vi "Connection Open.vi"(8 "error in (no error)":errorcluster, 11 "Connection Data In":T1) -> (0 "error out":errorcluster, 3 "Connection Data Out":T1)   [LabVIEW 2014, in "MSX-E3711_dll.lvlib"]
doc: "Abre la conexión del Web Server."
uses:
  MSX-E3711_dll.lvlib
  Typedef/Connection Data.ctl
  E:/Repositorio Magnis/INF002/v0/Modules/HAL/Drivers/Sync/ADDI-DATA MSX-E3711/API/MSXE371x.dll
  MSXE371x.dll
  E:/Repositorio Magnis/INF002/v0/Modules/HAL/Drivers/Sync/ADDI-DATA MSX-E3711/API/MXCommon.dll
  MXCommon.dll
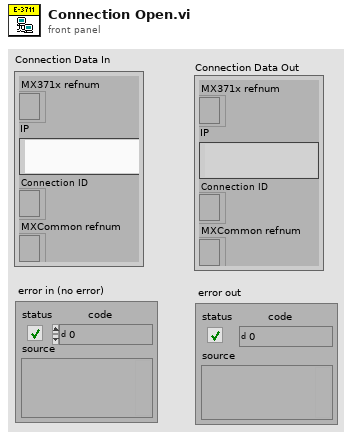
[diagram p1: front panel]
types:
  T1 = typedef "MSX-E3711_dll.lvlib/Connection Data.ctl" = cluster{"MX371x refnum":refnum<k24>, "IP":string, "Connection ID ":refnum<k5>, "MXCommon refnum":refnum<k24>}
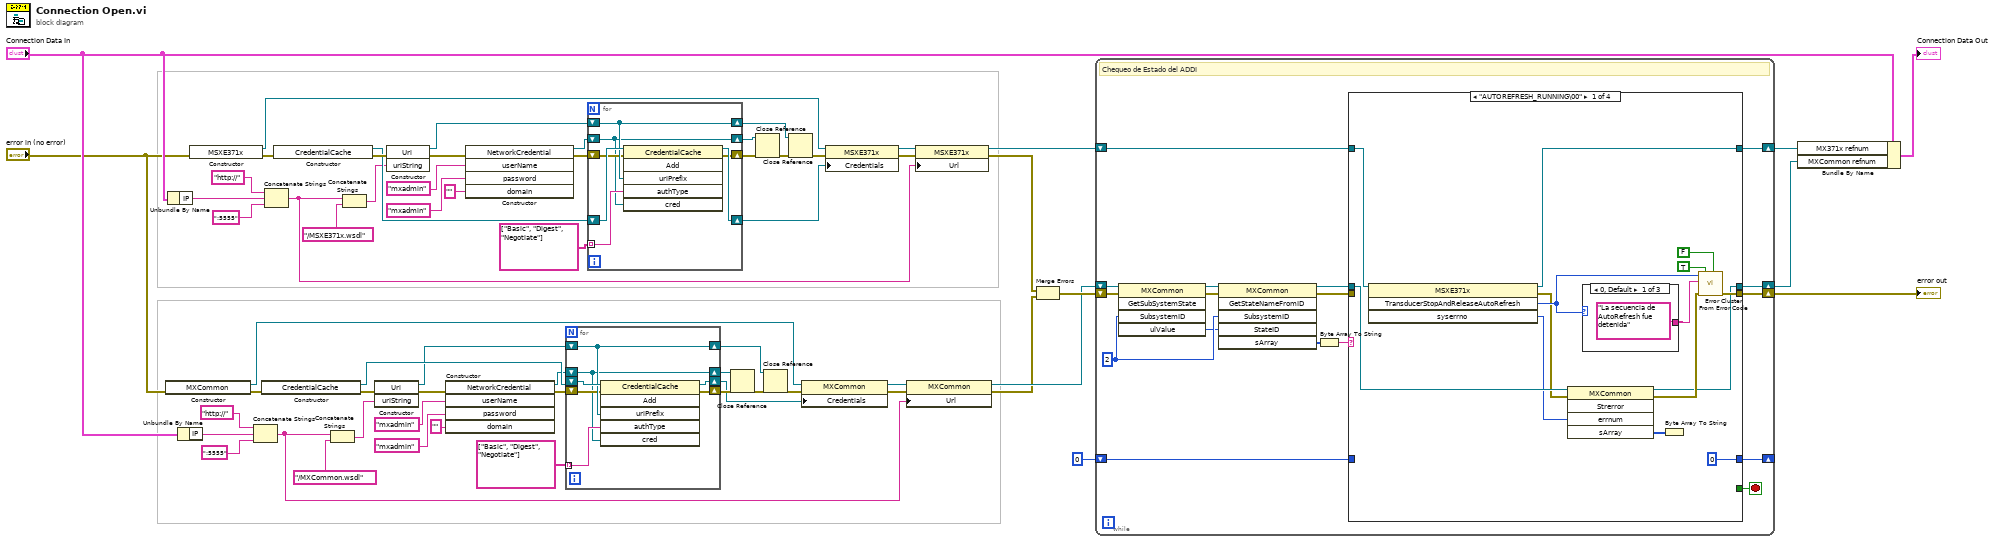
[diagram p0: block diagram]
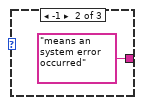
[diagram p2: hidden frame]
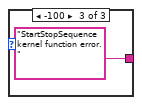
[diagram p3: hidden frame]
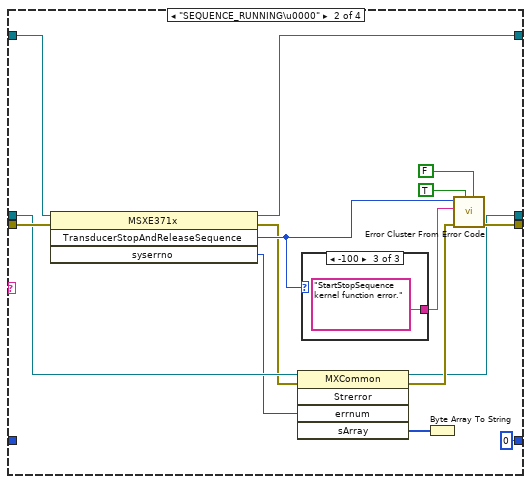
[diagram p4: hidden frame]
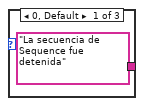
[diagram p5: hidden frame]
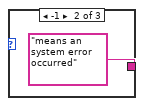
[diagram p6: hidden frame]
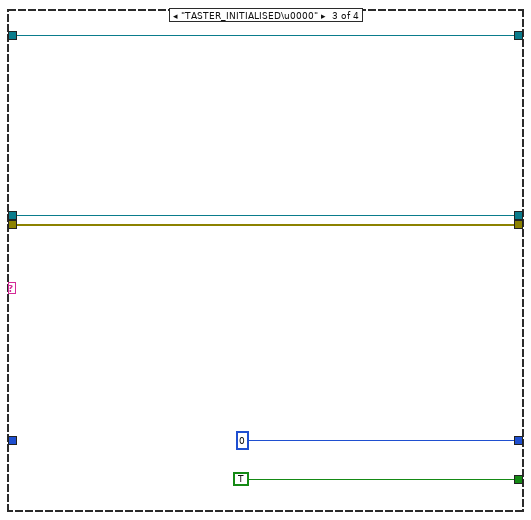
[diagram p7: hidden frame]
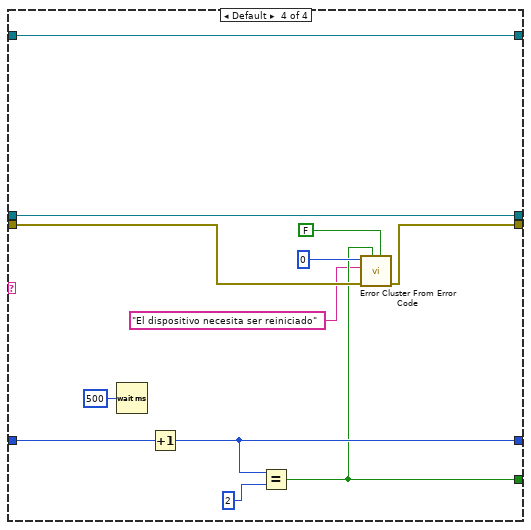
[diagram p8: hidden frame]
diagram:
  n1 = constructor class="MXCommon"(error in="error in (no error)") -> (reference out=w13:refnum<k24>, error out=w12:errorcluster)  [unwired: 2 in, 1 out]
  n2 = Unbundle By Name("Connection Data In") -> ("IP"=w45:string)
  n3 = Unbundle By Name("Connection Data In") -> ("IP"=w26:string)
  n4 = constructor class="MSXE371x"(error in="error in (no error)") -> (reference out=w5:refnum<k24>, error out=w11:errorcluster)  [unwired: 2 in, 1 out]
  n5 = Concatenate Strings("http://" ("string"), w26, ":5555" ("string")) -> (w17:string)
  n6 = constructor class="CredentialCache"(error in=w12) -> (reference out=w41:refnum<k24>, error out=w44:errorcluster)  [unwired: 2 in, 1 out]
  n7 = Concatenate Strings("http://" ("string"), w45, ":5555" ("string")) -> (w10:string)
  n8 = constructor class="CredentialCache"(error in=w11) -> (reference out=w61:refnum<k24>, error out=w64:errorcluster)  [unwired: 2 in, 1 out]
  n9 = Concatenate Strings(w17, "/MXCommon.wsdl" ("string")) -> (w28:string)
  n10 = Concatenate Strings(w10, "/MSXE371x.wsdl" ("string")) -> (w48:string)
  n11 = constructor class="Uri"(error in=w44, "uriString"=w28) -> (reference out=w40:refnum<k24>, error out=w43:errorcluster)  [unwired: 2 in, 2 out]
  n12 = constructor class="Uri"(error in=w64, "uriString"=w48) -> (reference out=w60:refnum<k24>, error out=w63:errorcluster)  [unwired: 2 in, 2 out]
  n13 = constructor class="NetworkCredential"(error in=w43, "userName"="mxadmin", "password"="mxadmin" ("userName"), "domain"="" ("userName")) -> (reference out=w39:refnum<k24>, error out=w38:errorcluster)  [unwired: 2 in, 4 out]
  n14 = constructor class="NetworkCredential"(error in=w63, "userName"="mxadmin", "password"="mxadmin" ("userName"), "domain"="" ("userName")) -> (reference out=w59:refnum<k24>, error out=w58:errorcluster)  [unwired: 2 in, 4 out]
  n15 = for {
    tunnel: string[] ["Basic", "Digest", "Negotiate"] -> [w66] mode=indexing
    shift-right: [w67] -> w34
    shift-left: w38 -> [w68]
    shift-right: [w70] -> w36
    shift-left: w40 -> [w70]
    shift-right: [w69] -> w20
    shift-left: w41 -> [w71]
    shift-right: [w65] -> w37
    shift-left: w39 -> [w65]
    n16 = invoke class="CredentialCache" method="Add"(reference=w71, error in=w68, "uriPrefix"=w70, "authType"=w66, "cred"=w65) -> (reference out=w69:refnum<k24>, error out=w67:errorcluster)  [unwired: 1 in, 4 out]
  }
  n17 = for {
    tunnel: string[] ["Basic", "Digest", "Negotiate"] -> [w73] mode=indexing
    shift-right: [w74] -> w54
    shift-left: w58 -> [w75]
    shift-right: [w77] -> w56
    shift-left: w60 -> [w77]
    shift-right: [w76] -> w3
    shift-left: w61 -> [w78]
    shift-right: [w72] -> w57
    shift-left: w59 -> [w72]
    n18 = invoke class="CredentialCache" method="Add"(reference=w78, error in=w75, "uriPrefix"=w77, "authType"=w73, "cred"=w72) -> (reference out=w76:refnum<k24>, error out=w74:errorcluster)  [unwired: 1 in, 4 out]
  }
  n19 = Close Reference(reference=w37, error in (no error)=w34) -> (error out=w35:errorcluster)
  n20 = Close Reference(reference=w57, error in (no error)=w54) -> (error out=w55:errorcluster)
  n21 = Close Reference(reference=w36, error in (no error)=w35) -> (error out=w14:errorcluster)
  n22 = Close Reference(reference=w56, error in (no error)=w55) -> (error out=w4:errorcluster)
  n23 = property class="MXCommon"(reference=w13, error in=w14, "Credentials"=w20) -> (reference out=w15:refnum<k24>, error out=w16:errorcluster)
  n24 = property class="MSXE371x"(reference=w5, error in=w4, "Credentials"=w3) -> (reference out=w7:refnum<k24>, error out=w6:errorcluster)
  n25 = property class="MXCommon"(reference=w15, error in=w16, "Url"=w17) -> (reference out=w19:refnum<k24>, error out=w18:errorcluster)
  n26 = property class="MSXE371x"(reference=w7, error in=w6, "Url"=w10) -> (reference out=w9:refnum<k24>, error out=w8:errorcluster)
  n27 = Merge Errors(w8, w18) -> (w24:errorcluster)
  n28 = while {
    shift-right: [w91] -> _
    shift-left: u32 0 ("milliseconds to wait") -> [w92]
    shift-right: [w90] -> w22
    shift-left: w19 -> [w87]
    shift-right: [w89] -> w21
    shift-left: w9 -> [w94]
    shift-right: [w88] -> w2
    shift-left: w24 -> [w86]
    stop <- w93 stop-if-true
    w85 = u64 2 ("SubsystemID 2")
    # "Chequeo de Estado del ADDI"
    n29 = invoke class="MXCommon" method="GetSubSystemState"(reference=w87, error in=w86, "SubsystemID"=w85) -> (reference out=w82:refnum<k24>, error out=w83:errorcluster, "ulValue"=w84:u64)  [unwired: 2 in, 2 out]
    n30 = invoke class="MXCommon" method="GetStateNameFromID"(reference=w82, error in=w83, "SubsystemID"=w85, "StateID"=w84) -> (reference out=w81:refnum<k24>, error out=w80:errorcluster, "sArray"=w79:u8[])  [unwired: 2 in, 3 out]
    n31 = Byte Array To String(unsigned byte array=w79) -> (string=w95:string)
    n32 = case shown="\"AUTOREFRESH_RUNNING\\00\"" w95 {
      tunnel: w94 -> [w104 w122 w131 w142]
      tunnel: w81 -> [w101 w118 w133 w143]
      tunnel: [_ _ TRUE w137] -> w93
      tunnel: w92 -> [_ _ _ w145]
      tunnel: [u32 0 u32 0 u32 0 w144] -> w91
      tunnel: [w97 w114 w133 w143] -> w90
      tunnel: [w103 w120 w131 w142] -> w89
      tunnel: w80 -> [_ w121 w132 w140]
      tunnel: [w105 w123 w132 w139] -> w88
      frame "AUTOREFRESH_RUNNING\u0000" {
        n33 = invoke class="MSXE371x" method="TransducerStopAndReleaseAutoRefresh"(reference=w104) -> (reference out=w103:refnum<k24>, error out=w100:errorcluster, "TransducerStopAndReleaseAutoRefresh"=w102:i32, "syserrno"=w99:i32)  [unwired: 3 in]
        n34 = invoke class="MXCommon" method="Strerror"(reference=w101, error in=w100, "errnum"=w99) -> (reference out=w97:refnum<k24>, error out=w98:errorcluster, "sArray"=w96:u8[])  [unwired: 2 in, 2 out]
        n35 = case shown="0, Default" w102 {
          tunnel: ["La secuencia de AutoRefresh fue detenida" "means an system error occurred" "StartStopSequence kernel function error."] -> w108
          frame 0, Default {
          }
          frame -1 {
          }
          frame -100 {
          }
        }
        n36 = Byte Array To String(unsigned byte array=w96) -> ()  [unwired: 1 out]
        n37 = call <vilib>:"Error Cluster From Error Code.vi"("is warning? (False)"=FALSE, "show call chain? (False)"=TRUE, "error in (no error)"=w98, "error message (\"\")"=w108, "error code (0)"=w102) -> ("error out"=w105:errorcluster)  [unwired: 4 in]
      }
      frame "SEQUENCE_RUNNING\u0000" {
        n38 = invoke class="MSXE371x" method="TransducerStopAndReleaseSequence"(reference=w122, error in=w121) -> (reference out=w120:refnum<k24>, error out=w117:errorcluster, "TransducerStopAndReleaseSequence"=w119:i32, "syserrno"=w116:i32)  [unwired: 2 in]
        n39 = invoke class="MXCommon" method="Strerror"(reference=w118, error in=w117, "errnum"=w116) -> (reference out=w114:refnum<k24>, error out=w115:errorcluster, "sArray"=w113:u8[])  [unwired: 2 in, 2 out]
        n40 = case shown="-100" w119 {
          tunnel: ["La secuencia de Sequence fue detenida" "means an system error occurred" "StartStopSequence kernel function error."] -> w126
          frame 0, Default {
          }
          frame -1 {
          }
          frame -100 {
          }
        }
        n41 = Byte Array To String(unsigned byte array=w113) -> ()  [unwired: 1 out]
        n42 = call <vilib>:"Error Cluster From Error Code.vi"("is warning? (False)"=FALSE, "show call chain? (False)"=TRUE, "error in (no error)"=w115, "error message (\"\")"=w126, "error code (0)"=w119) -> ("error out"=w123:errorcluster)  [unwired: 4 in]
      }
      frame "TASTER_INITIALISED\u0000" {
      }
      frame Default {
        n43 = Wait (ms)(milliseconds to wait=u32 500) -> ()  [unwired: 1 out]
        n44 = Increment(x=w145) -> (x+1=w144:u32)
        n45 = Equal?(x=w144, y=u32 2 ("milliseconds to wait")) -> (x = y?=w137:bool)
        n46 = call <vilib>:"Error Cluster From Error Code.vi"("is warning? (False)"=FALSE, "show call chain? (False)"=w137, "error in (no error)"=w140, "error message (\"\")"="El dispositivo necesita ser reiniciado", "error code (0)"=0) -> ("error out"=w139:errorcluster)  [unwired: 4 in]
      }
    }
  }
  "error out" <- w2
  n47 = Bundle By Name(cluster="Connection Data In", "MX371x refnum"=w21, "MXCommon refnum"=w22) -> (→"Connection Data Out":T1)
